vi "Main.vi"() -> ()   [LabVIEW 2019]
panel:
  in  "Update":bool
  in  "Element to Update":enum16{"<None>", "Name", "Age", "Is Married?"}(ring)=enum."Age"
  in  "Stop":bool
  in  "Is Married?":bool
  in  "Age":u8=23
  in  "Name":string="Adam"
  # "Data to Update"
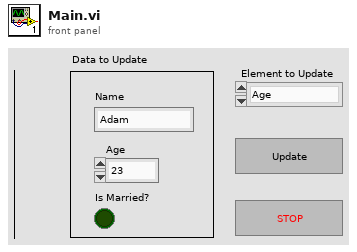
[diagram p1: front panel]
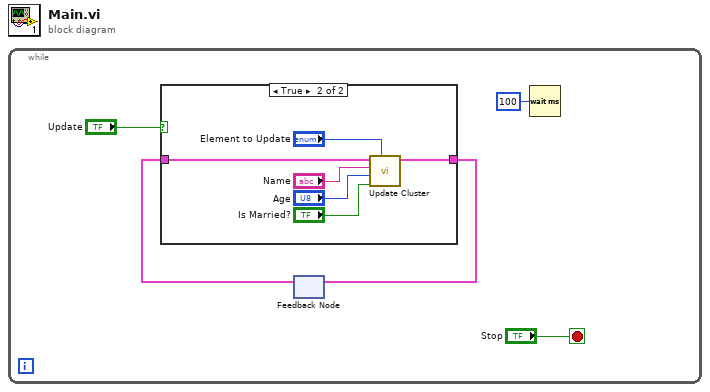
[diagram p0: block diagram]
diagram:
  n1 = while {
    stop <- "Stop" stop-if-true
    n2 = feedback #1() -> (w2:cluster{})  [unwired: 1 in]
    n3 = case shown="True" "Update" {
      tunnel: [w6 w8] -> w3
      tunnel: w2 -> [w6 w7]
      frame False {
      }
      frame True {
        n4 = call "Update Cluster.vi"("Element to Update"="Element to Update", "Is Married?"="Is Married?", "Age"="Age", "Name"="Name", "Customer Data in"=w7) -> ("Customer Data out"=w8:cluster{})  [unwired: 6 in]
      }
    }
    n5 = feedback-in #1(w3) -> ()
    n6 = Wait (ms)(milliseconds to wait=u32 100) -> ()  [unwired: 1 out]
  }
